vi "Teleop.vi"(10 "Match Info":T1={"Autonomous Elapsed Seconds"=0.0, "TeleOp Elapsed Seconds"=0.0, "Disabled Elapsed Seconds"=0.0, "Visited Autonomous"=FALSE, "Visited TeleOp"=FALSE, "Visited Disabled"=FALSE, "Autonomous Settings"={"Autonomous Style"=enum."Independent", "VI Refnum"=refnum}}, 11 "Call Context":T2) -> ()   [LabVIEW 2019]
doc: "This VI is called for each TeleOp packet received from the DS where the robot is not disabled. It is often used to read from the joysticks and update I/O or to update setpoints for timed control loops. It should complete and return within 20 milliseconds or it may miss DS packets."
uses:
  <vilib>/Rock Robotics/WPI/DriverStation/WPI_DriverStationDerivedRobotMode.ctl
  <vilib>/Rock Robotics/WPI/DriverStation/WPI_DriverStationMatch Info.ctl
  <vilib>/Rock Robotics/WPI/Utilities/WPI_GetSetVariantRefNum.vi
  <vilib>/Rock Robotics/Network Tables/NT Read Number.vi
  Robot Global Data.vi
  <vilib>/Rock Robotics/Network Tables/NT Write Number.vi
panel:
  # "Click here to set min"
  # "Click here to set max"
  # "Click here to set min"
  # "Click here to set max"
  # "Click here to set min"
  # "Click here to set max"
  # "Click here to set min"
  # "Click here to set max"
  # "Click here to set min"
  # "Click here to set max"
  # "Click here to set min"
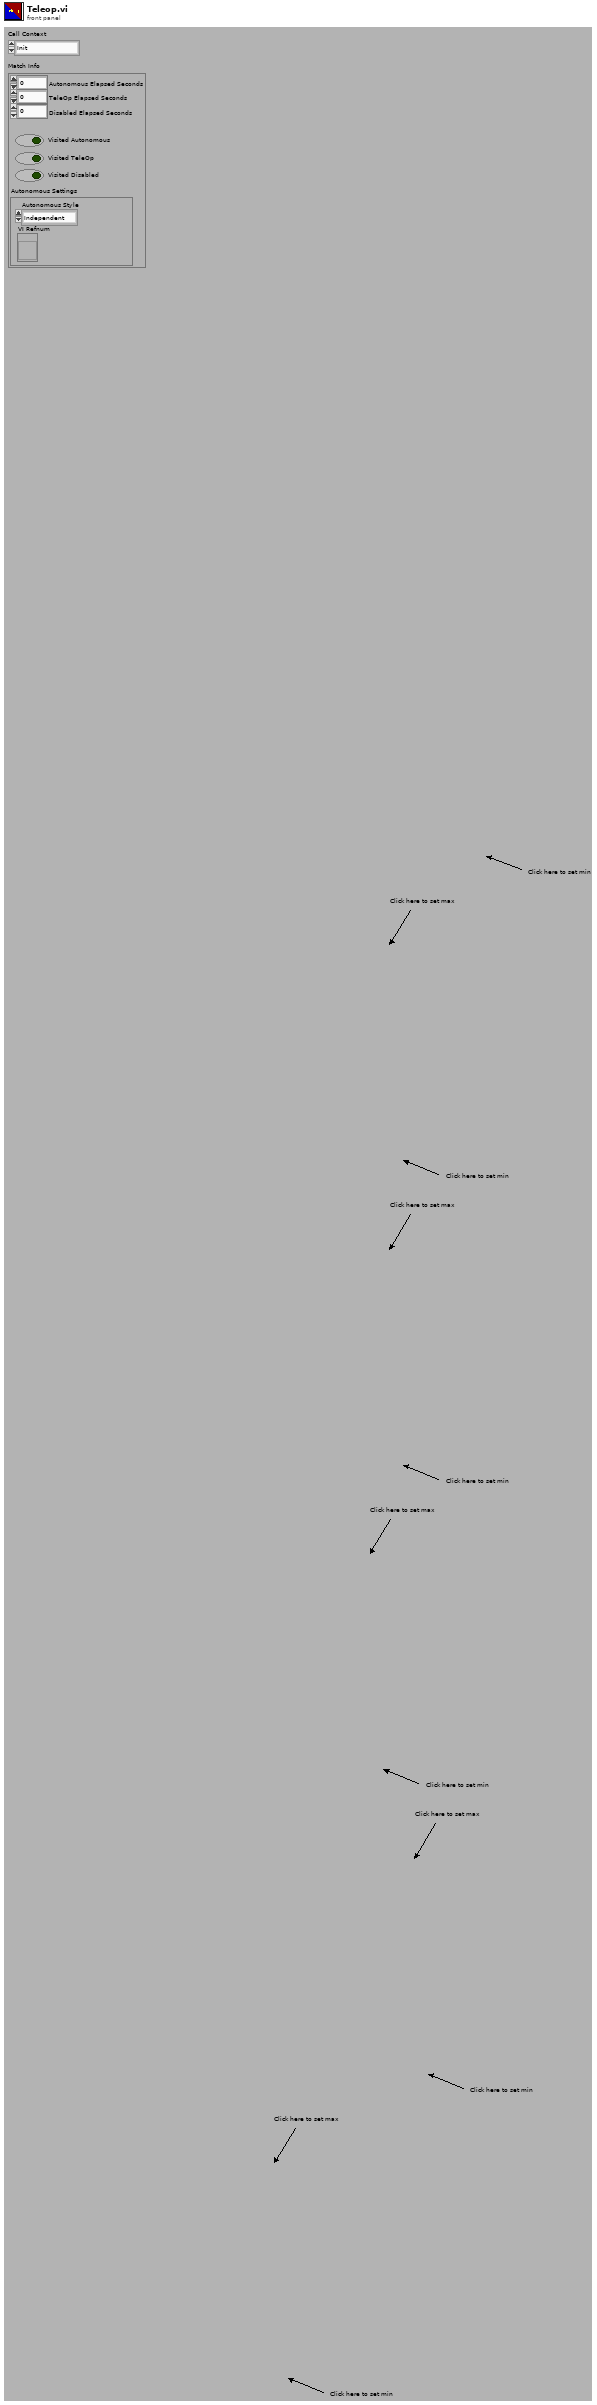
[diagram p1: front panel]
types:
  T1 = typedef "WPI_DriverStationMatch Info.ctl" = cluster{"Autonomous Elapsed Seconds":dbl, "TeleOp Elapsed Seconds":dbl, "Disabled Elapsed Seconds":dbl, "Visited Autonomous":bool, "Visited TeleOp":bool, "Visited Disabled":bool, "Autonomous Settings":cluster{"Autonomous Style":enum16{"Iterative", "Independent"}, "VI Refnum":refnum<vi>}}
  T2 = typedef "WPI_DriverStationDerivedRobotMode.ctl" = enum16{"Init", "Execute", "Stop"}
  T3 = typedef "WPI_MotorControlDeviceRef.ctl" = cluster{"DeviceStatus":errorcluster, "Type":T4, "PWM":cluster{"PWM Channel":T5, "DeadBand":T6}, "CAN":cluster{"Device Number":u8, "SetOutput VI Ref":variant, "GetOutput VI Ref":variant, "Enable VI Ref":variant, "Disable VI Ref":variant, "Data":variant}, "Invert":bool, "DIO PWM":cluster{"PWM \"Enable\" Channel":T5, "DIOChannel":T7, "PWM Rate":dbl}}
  T4 = typedef "WPI_MotorControlType.ctl" = enum16{"PWM", "CAN", "DIO PWM"}
  T5 = typedef "FPGA_DIOPWMChannel.ctl" = enum8{"PWM 0", "PWM 1", "PWM 2", "PWM 3", "PWM 4", "PWM 5", "PWM 6", "PWM 7", "PWM 8", "PWM 9", "PWM MXP 0", "PWM MXP 1", "PWM MXP 2", "PWM MXP 3", "PWM MXP 4", "PWM MXP 5", "PWM MXP 6", "PWM MXP 7", "PWM MXP 8", "PWM MXP 9", "Invalid"}
  T6 = typedef "WPI_PWMDeadband.ctl" = cluster{"Name":string, "maxPositivePwm":i32, "minPositivePwm":i32, "centerPwm":i32, "maxNegativePwm":i32, "minNegativePwm":i32, "angularRange":u16}
  T7 = typedef "FPGA_DIOChannel.ctl" = enum8{"DIO 0", "DIO 1", "DIO 2", "DIO 3", "DIO 4", "DIO 5", "DIO 6", "DIO 7", "DIO 8", "DIO 9", "DIO MXP 0", "DIO MXP 1", "DIO MXP 2", "DIO MXP 3", "DIO MXP 4", "DIO MXP 5", "DIO MXP 6", "DIO MXP 7", "DIO MXP 8", "DIO MXP 9", "DIO MXP 10", "DIO MXP 11", "DIO MXP 12", "DIO MXP 13", "DIO MXP 14", "DIO MXP 15", "SPI Port CS1", "SPI Port CS2", "SPI Port CS3", "SPI Port MISO", "SPI Port MOSI", "Invalid"}
  T8 = typedef "WPI_JoystickDevRef.ctl" = cluster{"Device":T9}
  T9 = typedef "WPI_JoystickDeviceEnum.ctl" = enum16{"USB 0", "USB 1", "USB 2", "USB 3", "USB 4", "USB 5"}
  T10 = typedef "WPI_RobotDriveDevRef.ctl" = cluster{"DevStatus":errorcluster, "Motors[]":T3[], "Square Inputs":bool, "Max Output":dbl}
  T11 = cluster{"JoystickDevRef":T8, "RobotDriveDevRef":T10}
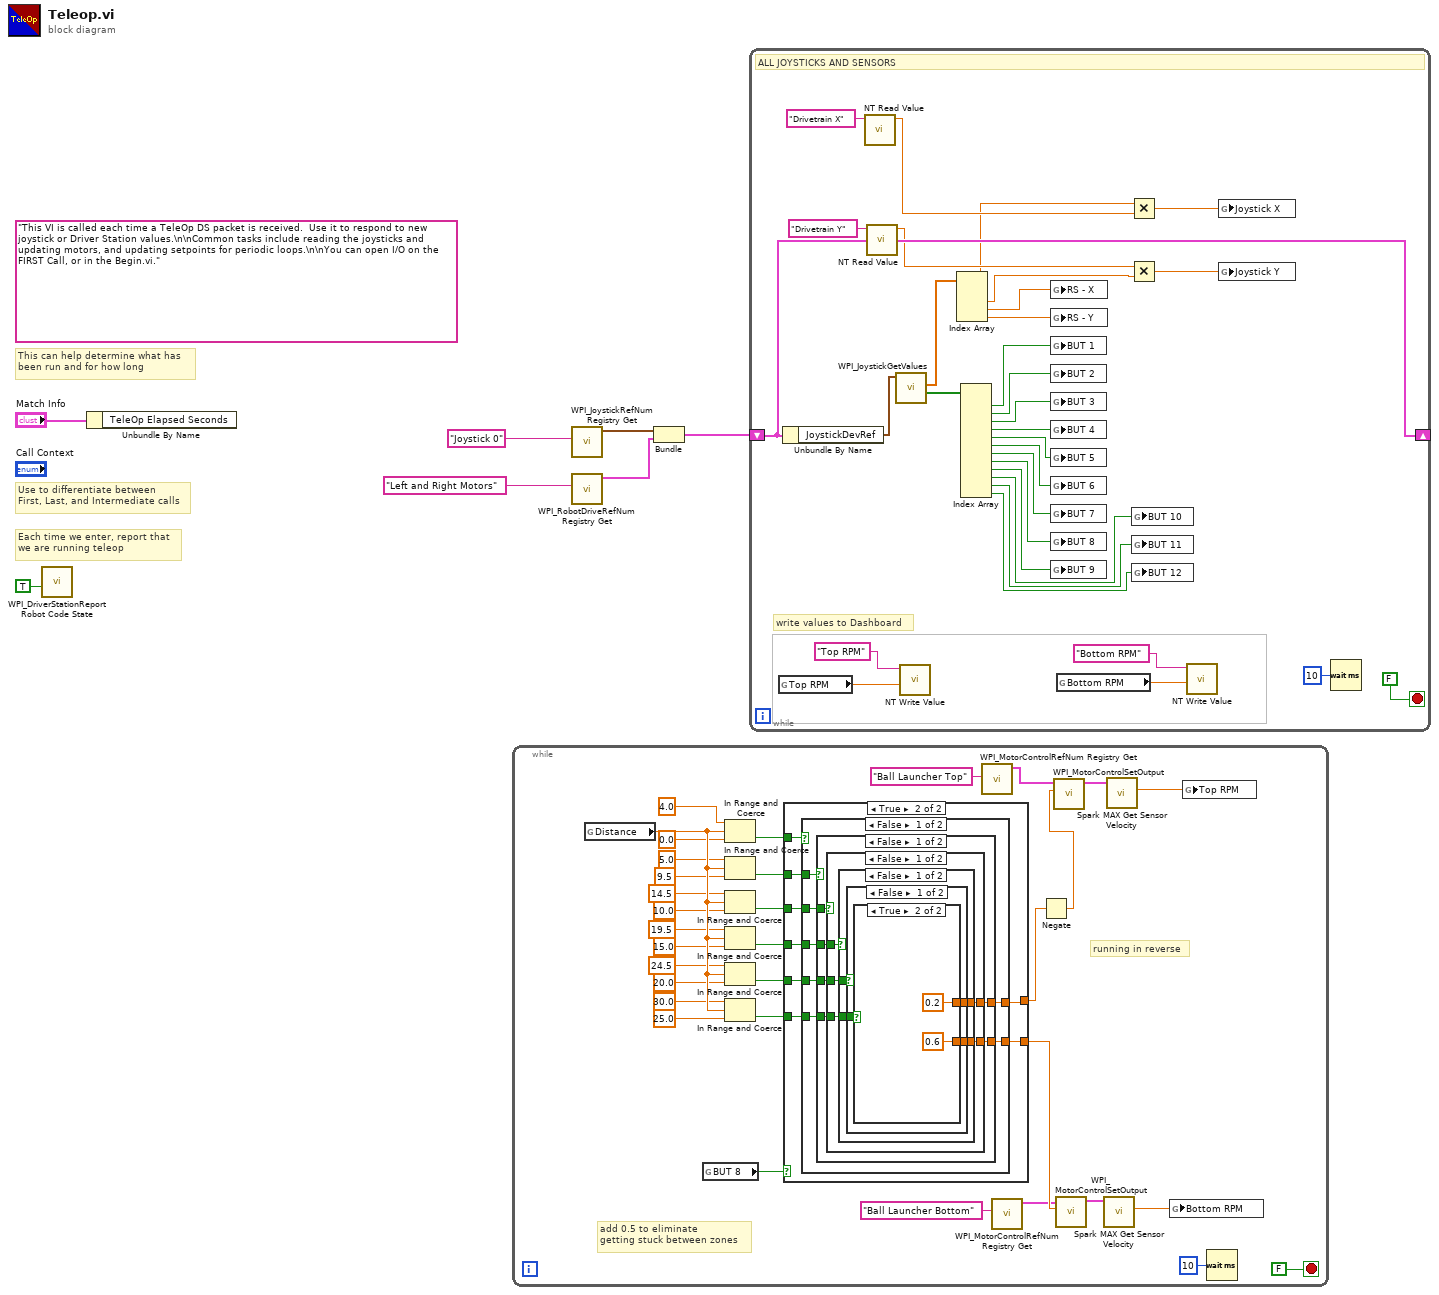
[diagram p0: block diagram]
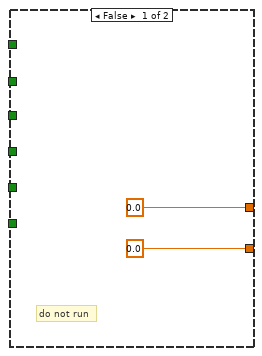
[diagram p2: hidden frame]
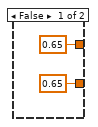
[diagram p3: hidden frame]
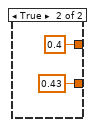
[diagram p4: hidden frame]
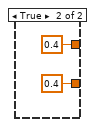
[diagram p5: hidden frame]
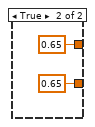
[diagram p6: hidden frame]
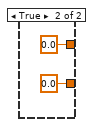
[diagram p7: hidden frame]
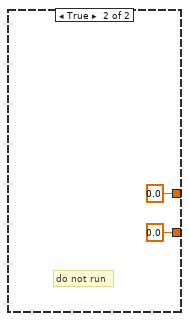
[diagram p8: hidden frame]
diagram:
  (unwired) "This VI is called each time a TeleOp DS packet is received.  Use it to respond to new joystick or Driver Station values.\n\nCommon tasks include reading the joysticks and updating motors, and updating setpoints for periodic loops.\n\nYou can open I/O on the FIRST Call, or in the Begin.vi."
  # "Each time we enter, report that\nwe are running teleop"
  # "Use to differentiate between\nFirst, Last, and Intermediate calls"
  # "This can help determine what has\nbeen run and for how long"
  n1 = call <vilib>:"WPI_DriverStationReport Robot Code State.vi"("TeleOp"=TRUE ("Autonomous")) -> ()  [unwired: 10 in, 1 out]
  n2 = Unbundle By Name("Match Info") -> ()  [unwired: 1 out]
  n3 = while {
    stop <- FALSE stop-if-true
    # "running in reverse"
    # "add 0.5 to eliminate\ngetting stuck between zones"
    n4 = global read "Robot Global Data.vi" "Distance"() -> (w40:dbl)
    n5 = global read "Robot Global Data.vi" "BUT 8"() -> (w18:bool)
    n6 = In Range and Coerce(upper limit=4.0, x=w40, lower limit=0.0) -> (In Range?=w37:bool)  [unwired: 1 out]
    n7 = In Range and Coerce(upper limit=5.0, x=w40, lower limit=9.5) -> (In Range?=w36:bool)  [unwired: 1 out]
    n8 = In Range and Coerce(upper limit=14.5, x=w40, lower limit=10.0) -> (In Range?=w20:bool)  [unwired: 1 out]
    n9 = In Range and Coerce(upper limit=19.5, x=w40, lower limit=15.0) -> (In Range?=w21:bool)  [unwired: 1 out]
    n10 = In Range and Coerce(upper limit=24.5, x=w40, lower limit=20.0) -> (In Range?=w22:bool)  [unwired: 1 out]
    n11 = In Range and Coerce(upper limit=30.0, x=w40, lower limit=25.0) -> (In Range?=w23:bool)  [unwired: 1 out]
    n12 = case shown="True" w18 {
      tunnel: [0.0 ("Output") w44] -> w39
      tunnel: [0.0 ("Output") w43] -> w19
      tunnel: w37 -> [_ w50]
      tunnel: w20 -> [_ w48]
      tunnel: w21 -> [_ w47]
      tunnel: w22 -> [_ w46]
      tunnel: w23 -> [_ w45]
      tunnel: w36 -> [_ w49]
      frame False {
        # "do not run"
      }
      frame True {
        n13 = case shown="False" w50 {
          tunnel: w49 -> [w57 _]
          tunnel: w48 -> [w56 _]
          tunnel: w47 -> [w55 _]
          tunnel: w46 -> [w54 _]
          tunnel: w45 -> [w53 _]
          tunnel: [w52 0.0 ("Output")] -> w44
          tunnel: [w51 0.0 ("Output")] -> w43
          frame False {
            n14 = case shown="False" w57 {
              tunnel: w56 -> [w63 _]
              tunnel: w55 -> [w62 _]
              tunnel: w54 -> [w61 _]
              tunnel: w53 -> [w60 _]
              tunnel: [w59 0.0 ("Output")] -> w52
              tunnel: [w58 0.0 ("Output")] -> w51
              frame False {
                n15 = case shown="False" w63 {
                  tunnel: w62 -> [w68 _]
                  tunnel: w61 -> [w67 _]
                  tunnel: w60 -> [w66 _]
                  tunnel: [w65 0.65 ("Output")] -> w59
                  tunnel: [w64 0.65 ("Output")] -> w58
                  frame False {
                    n16 = case shown="False" w68 {
                      tunnel: w67 -> [w72 _]
                      tunnel: w66 -> [w71 _]
                      tunnel: [w70 0.4 ("Output")] -> w65
                      tunnel: [w69 0.4 ("Output")] -> w64
                      frame False {
                        n17 = case shown="False" w72 {
                          tunnel: w71 -> [w75 _]
                          tunnel: [w74 0.4 ("Output")] -> w70
                          tunnel: [w73 0.43 ("Output")] -> w69
                          frame False {
                            n18 = case shown="True" w75 {
                              tunnel: [0.65 ("Output") 0.2 ("Output")] -> w74
                              tunnel: [0.65 ("Output") 0.6 ("Output")] -> w73
                              frame False {
                              }
                              frame True {
                              }
                            }
                          }
                          frame True {
                          }
                        }
                      }
                      frame True {
                      }
                    }
                  }
                  frame True {
                  }
                }
              }
              frame True {
              }
            }
          }
          frame True {
            # "do not run"
          }
        }
      }
    }
    n19 = call <vilib>:"WPI_MotorControlRefNum Registry Get.vi"("refnum name"="Ball Launcher Top") -> ("MotorControlDevRef"=w13:T3)  [unwired: 9 in, 1 out]
    n20 = call <vilib>:"WPI_MotorControlRefNum Registry Get.vi"("refnum name"="Ball Launcher Bottom") -> ("MotorControlDevRef"=w11:T3)  [unwired: 9 in, 1 out]
    n21 = Negate(x=w39) -> (-x=w38:dbl)
    n22 = call <vilib>:"WPI_MotorControlSetOutput.vi"("Output"=w38, "MotorControlDevRef"=w13) -> ("MotorControlDevRef"=w16:T3)  [unwired: 7 in, 2 out]
    n23 = call <vilib>:"WPI_MotorControlSetOutput.vi"("Output"=w19, "MotorControlDevRef"=w11) -> ("MotorControlDevRef"=w17:T3)  [unwired: 7 in, 2 out]
    n24 = call <vilib>:"Spark MAX Get Sensor Velocity.vi"("MotorControlDevRef in"=w17) -> ("Sensor Velocity"=w15:dbl)  [unwired: 7 in, 3 out]
    n25 = call <vilib>:"Spark MAX Get Sensor Velocity.vi"("MotorControlDevRef in"=w16) -> ("Sensor Velocity"=w14:dbl)  [unwired: 7 in, 3 out]
    n26 = global write "Robot Global Data.vi" "Bottom RPM"(w15) -> ()
    n27 = global write "Robot Global Data.vi" "Top RPM"(w14) -> ()
    n28 = Wait (ms)(milliseconds to wait=u32 10) -> ()  [unwired: 1 out]
  }
  n29 = call <vilib>:"WPI_JoystickRefNum Registry Get.vi"("refnum name"="Joystick 0") -> ("JoystickDevRef"=w3:T8)  [unwired: 1 in, 9 out]
  n30 = call <vilib>:"WPI_RobotDriveRefNum Registry Get.vi"("refnum name"="Left and Right Motors") -> ("RobotDriveDevRef"=w2:T10)  [unwired: 1 in, 9 out]
  n31 = Bundle("JoystickDevRef"=w3, "RobotDriveDevRef"=w2) -> (w1:T11)  [unwired: 1 out]
  n32 = while {
    shift-right: [w106] -> _
    shift-left: w1 -> [w106]
    stop <- FALSE stop-if-true
    # "write values to Dashboard"
    # "ALL JOYSTICKS AND SENSORS"
    n33 = global read "Robot Global Data.vi" "Top RPM"() -> (w100:dbl)
    n34 = Unbundle By Name(w106) -> ("JoystickDevRef"=w120:T8)
    n35 = call-poly <vilib>:"NT Read Value.vi"("Name"="Drivetrain X") -> ("Numeric"=w94:dbl)  [unwired: 9 in, 1 out]
    n36 = call-poly <vilib>:"NT Read Value.vi"("Name"="Drivetrain Y") -> ("Numeric"=w95:dbl)  [unwired: 9 in, 1 out]
    n37 = call <vilib>:"WPI_JoystickGetValues.vi"("JoystickDevRef"=w120) -> ("Buttons"=w119:bool[], "Axes"=w105:dbl[])  [unwired: 6 in, 3 out]
    n38 = call-poly <vilib>:"NT Write Value.vi"("Numeric"=w100, "Name"="Top RPM") -> ()  [unwired: 9 in, 1 out]
    n39 = Index Array(array=w105) -> (element #1=w91:dbl, element #2=w90:dbl, element #3=w92:dbl, element #4=w103:dbl)  [unwired: 4 in]
    n40 = Index Array(array=w119) -> (element #1=w118:bool, element #2=w117:bool, element #3=w116:bool, element #4=w115:bool, element #5=w114:bool, element #6=w113:bool, element #7=w112:bool, element #8=w111:bool, element #9=w110:bool, element #10=w109:bool, element #11=w108:bool, element #12=w107:bool)  [unwired: 12 in]
    n41 = global write "Robot Global Data.vi" "RS - X"(w92) -> ()
    n42 = global write "Robot Global Data.vi" "RS - Y"(w103) -> ()
    n43 = global write "Robot Global Data.vi" "BUT 1"(w118) -> ()
    n44 = global write "Robot Global Data.vi" "BUT 2"(w117) -> ()
    n45 = global write "Robot Global Data.vi" "BUT 3"(w116) -> ()
    n46 = global write "Robot Global Data.vi" "BUT 4"(w115) -> ()
    n47 = global write "Robot Global Data.vi" "BUT 5"(w114) -> ()
    n48 = global write "Robot Global Data.vi" "BUT 6"(w113) -> ()
    n49 = global write "Robot Global Data.vi" "BUT 7"(w112) -> ()
    n50 = global write "Robot Global Data.vi" "BUT 8"(w111) -> ()
    n51 = global write "Robot Global Data.vi" "BUT 9"(w110) -> ()
    n52 = global read "Robot Global Data.vi" "Bottom RPM"() -> (w98:dbl)
    n53 = Multiply(x=w91, y=w94) -> (x*y=w93:dbl)
    n54 = Multiply(x=w95, y=w90) -> (x*y=w104:dbl)
    n55 = global write "Robot Global Data.vi" "BUT 10"(w109) -> ()
    n56 = global write "Robot Global Data.vi" "BUT 11"(w108) -> ()
    n57 = global write "Robot Global Data.vi" "BUT 12"(w107) -> ()
    n58 = call-poly <vilib>:"NT Write Value.vi"("Numeric"=w98, "Name"="Bottom RPM") -> ()  [unwired: 9 in, 1 out]
    n59 = global write "Robot Global Data.vi" "Joystick X"(w93) -> ()
    n60 = global write "Robot Global Data.vi" "Joystick Y"(w104) -> ()
    n61 = Wait (ms)(milliseconds to wait=u32 10) -> ()  [unwired: 1 out]
  }
